vi "Drive Immediate.vi"(6 "Cluster":cluster{dbl, dbl, dbl, dbl, dbl, dbl}, 7 "Description":string, 8 "Command Info In":T1, 9 "Deadband Value":dbl=0.01, 10 "Right Setpoint":dbl, 11 "Left Setpoint":dbl) -> (0 "Command Info Out":T1)   [LabVIEW 2019]
doc: "Often used for joystick control, this VI checks to see that the joystick axes are outside the deadband and updates the motors appropriately."
uses:
  <vilib>/Rock Robotics/WPI/Framework/Command Status Info.ctl
  <vilib>/Rock Robotics/WPI/Framework/Completion Status.ctl
  <vilib>/Rock Robotics/WPI/Framework/Completion Notifier.ctl
  Implementation/Drive Setpoints.ctl
  Implementation/Drive Operations.ctl
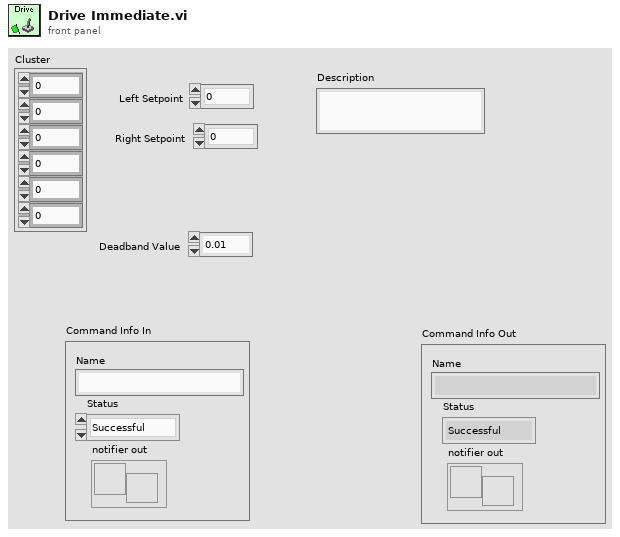
[diagram p1: front panel]
types:
  T1 = typedef "Command Status Info.ctl" = cluster{"Name":string, "Status":T2, "notifier out":T3}
  T2 = typedef "Completion Status.ctl" = enum16{"Successful", "Aborted", "Incomplete"}
  T3 = typedef "Completion Notifier.ctl" = refnum<notifier>
  T4 = typedef "Drive Setpoints.ctl" = cluster{"Operation":T5, "Left Setpoint":dbl, "Right Setpoint":dbl, "Duration":dbl, "left setpoint\nBack":dbl, "right setpoint\nBack":dbl, "left setpoint\nBack spin":dbl, "right setpoint\nBack spin":dbl, "left setpoint \nfront spin":dbl, "right setpoint\nfront spin":dbl}
  T5 = typedef "Drive Operations.ctl" = enum16{"Reserve", "Read Current", "Immediate", "Drive for Time", "Drive for Distance"}
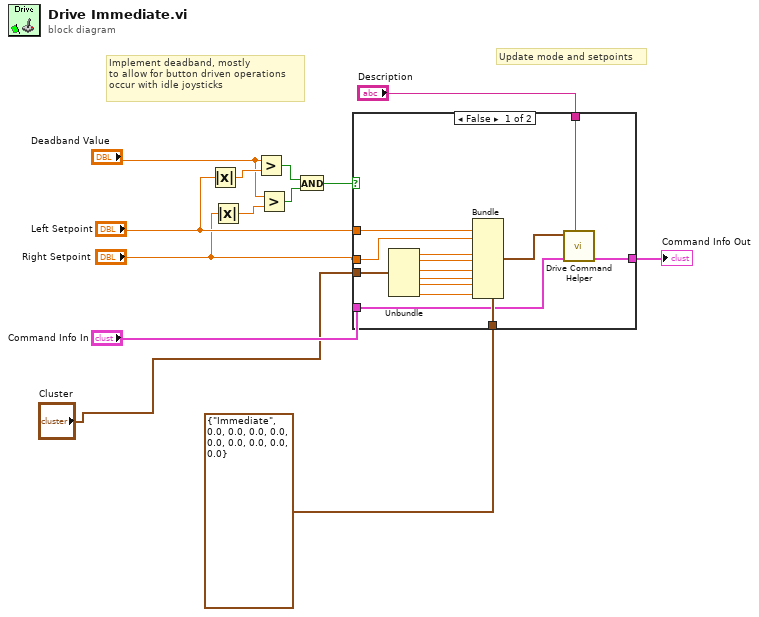
[diagram p0: block diagram]
diagram:
  # "Implement deadband, mostly\nto allow for button driven operations\noccur with idle joysticks"
  # "Update mode and setpoints"
  n1 = Absolute Value(x="Left Setpoint") -> (abs(x)=w13:dbl)
  n2 = Absolute Value(x="Right Setpoint") -> (abs(x)=w5:dbl)
  n3 = Greater?(x="Deadband Value", y=w13) -> (0:w7:bool)
  n4 = Greater?(x="Deadband Value", y=w5) -> (0:w3:bool)
  n5 = And(x=w7, y=w3) -> (x .and. y?=w6:bool)
  n6 = case shown="False" w6 {
    tunnel: "Left Setpoint" -> [w27 _]
    tunnel: T4 {"Operation"=enum."Immediate", "Left Setpoint"=0.0, "Right Setpoint"=0.0, "Duration"=0.0, "left setpoint\nBack"=0.0, "right setpoint\nBack"=0.0, "left setpoint\nBack spin"=0.0, "right setpoint\nBack spin"=0.0, "left setpoint \nfront spin"=0.0, "right setpoint\nfront spin"=0.0} ("SubSystem Data") -> [w26 _]
    tunnel: [w25 w28] -> w12
    tunnel: "Command Info In" -> [w24 w28]
    tunnel: "Description" -> [w22 _]
    tunnel: "Right Setpoint" -> [w21 _]
    tunnel: "Cluster" -> [w20 _]
    frame False {
      n7 = Unbundle(w20) -> (w19:dbl, w18:dbl, w17:dbl, w16:dbl, w15:dbl, w14:dbl)
      n8 = Bundle(cluster=w26, "Left Setpoint"=w27, "Right Setpoint"=w21, "left setpoint\nBack"=w19, "right setpoint\nBack"=w18, "left setpoint\nBack spin"=w17, "right setpoint\nBack spin"=w16, "left setpoint \nfront spin"=w15, "right setpoint\nfront spin"=w14) -> (w23:T4)  [unwired: 2 in]
      n9 = call "Drive Command Helper.vi"("Description"=w22, "Command Info In"=w24, "SubSystem Data"=w23) -> ("Command Info Out"=w25:T1)  [unwired: 6 in, 2 out]
    }
    frame True {
    }
  }
  "Command Info Out" <- w12
